vi "horn_coplanar.vi"(8 "Right points (world)":sgl[][](array[numeric]) format="%#.5f", 11 "Left points (lights)":sgl[][](array[numeric]) format="%#.5f") -> (2 "LR transform":T1)   [LabVIEW 2014]
uses:
  <vilib>/Analysis/Matrix/Datatypes/RealMatrix.ctl
  <vilib>/Analysis/baseanly.llb/Real Dot Product.vi
  <vilib>/Analysis/baseanly.llb/Real A x B.vi
  utilities/labview/norm_vec.vi
  <vilib>/Analysis/Matrix/Numeric/Conversions/Array To Matrix - RA.vi
  <vilib>/Analysis/NI_AALBase.lvlib
  <vilib>/Analysis/Matrix/NI_Matrix.lvlib
panel:
  # "Linear homogenous transform that maps the left points onto the right points."
  # "The input points, each row a point.   The points should be non-collinear and co-planar , which in practice only precisely applies when there are exactly three points.  This will give a reasonable result for > 3 points, but it will be not be a least-squares solution, being overly influenced by the first two points."
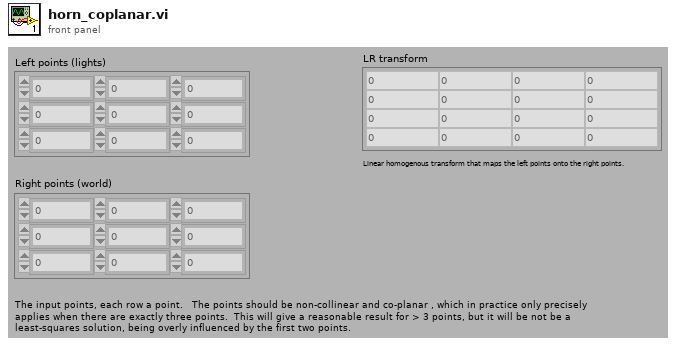
[diagram p1: front panel]
types:
  T1 = typedef "NI_Matrix.lvlib/RealMatrix.ctl" = dbl[][]
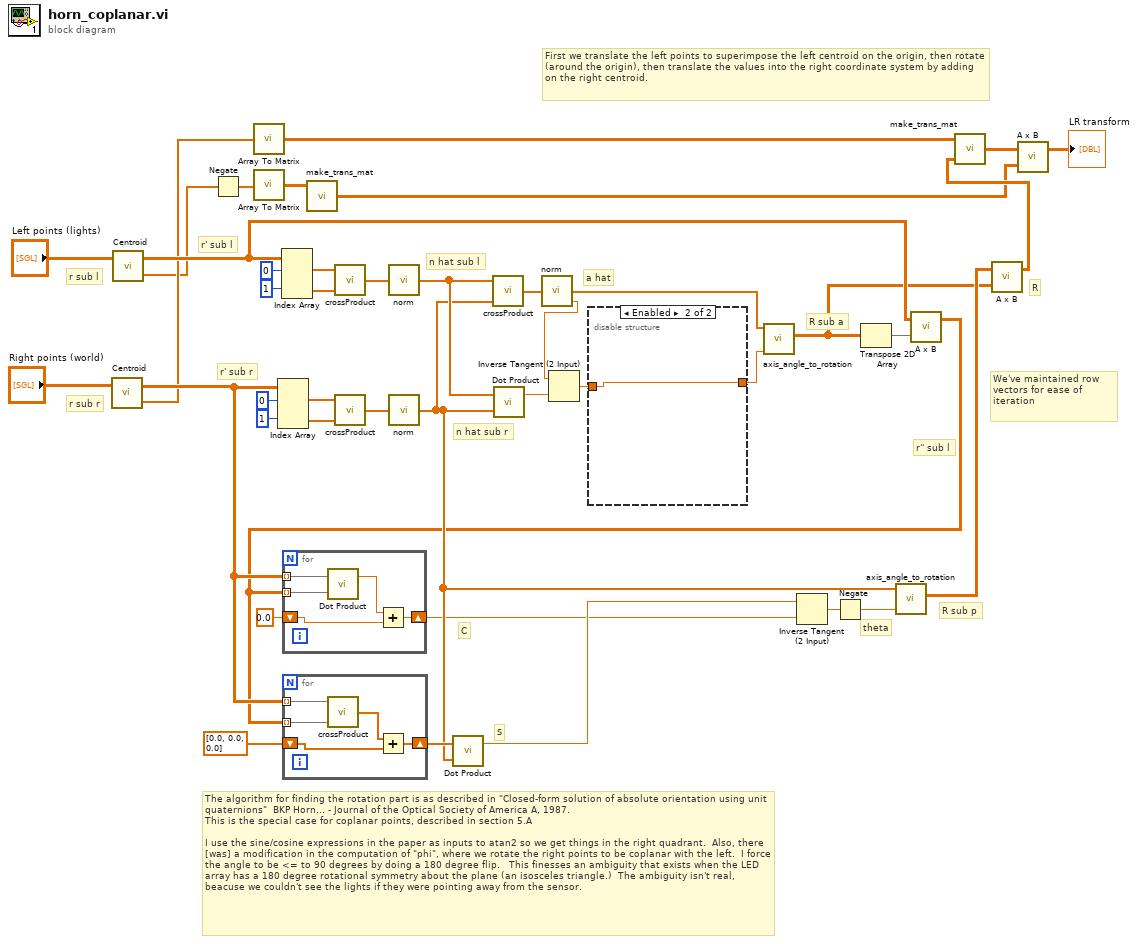
[diagram p0: block diagram]
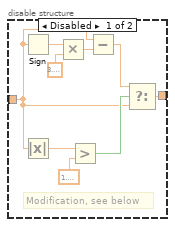
[diagram p2: hidden frame]
diagram:
  # "We've maintained row vectors for ease of iteration"
  # "First we translate the left points to superimpose the left centroid on the origin, then rotate (around the origin), then translate the values into the right coordinate system by adding on the right centroid."
  # "The algorithm for finding the rotation part is as described in \"Closed-form solution of absolute orientation using unit quaternions\"  BKP Horn… - Journal of the Optical Society of America A, 1987.\nThis is the special case for coplanar points, described in section 5.A\n\nI use the sine/cosine expressions in the paper as inputs to atan2 so we get things in the right quadrant.  Also, there [was] a modification in the computation of \"phi\", where we rotate the right points to be coplanar with the left.  I force the angle to be <= to 90 degrees by doing a 180 degree flip.   This finesses an ambiguity that exists when the LED array has a 180 degree rotational symmetry about the plane (an isosceles triangle.)  The ambiguity isn't real, beacuse we couldn't see the lights if they were pointing away from the sensor."
  # "R"
  # "R sub p"
  # "theta"
  # "S"
  # "C"
  # "r'' sub l"
  # "R sub a"
  # "r' sub r"
  # "r' sub l"
  # "r sub l"
  # "r sub r"
  # "a hat"
  # "n hat sub r"
  # "n hat sub l"
  n1 = call "Centroid.vi"("Points"="Right points (world)") -> ("Centroid"=w5:sgl[], "Offset vectors"=w24:sgl[][])  [unwired: 1 out]
  n2 = call "Centroid.vi"("Points"="Left points (lights)") -> ("Centroid"=w3:sgl[], "Offset vectors"=w26:sgl[][])  [unwired: 1 out]
  n3 = Negate(x=w3) -> (-x=w4:sgl[])
  n4 = call-poly <vilib>:"Array To Matrix.vi"("Real 1D Array"=w5) -> ("Real Matrix (Column Vector)"=w7:T1)
  n5 = call-poly <vilib>:"Array To Matrix.vi"("Real 1D Array"=w4) -> ("Real Matrix (Column Vector)"=w10:T1)
  n6 = Index Array(array=w24, index (row) #1=0 ("index"), index (row) #2=1 ("index")) -> (element #1=w32:sgl[], element #2=w31:sgl[])  [unwired: 2 in]
  n7 = Index Array(array=w26, index (row) #1=0 ("index"), index (row) #2=1 ("index")) -> (element #1=w38:sgl[], element #2=w37:sgl[])  [unwired: 2 in]
  n8 = call "make_trans_mat.vi"("Translation"=w10) -> ("Transform"=w8:T1)  [unwired: 1 in, 3 out]
  n9 = call "crossProduct.vi"("B"=w37, "A"=w38) -> ("A x B"=w36:dbl[])  [unwired: 3 out]
  n10 = call "crossProduct.vi"("B"=w31, "A"=w32) -> ("A x B"=w35:dbl[])  [unwired: 3 out]
  n11 = call-poly "norm.vi"("vector"=w36) -> ("normalized vector"=w29:dbl[])  [unwired: 4 out]
  n12 = call-poly "norm.vi"("vector"=w35) -> ("normalized vector"=w21:dbl[])  [unwired: 4 out]
  n13 = call "crossProduct.vi"("B"=w21, "A"=w29) -> ("A x B"=w30:dbl[])  [unwired: 3 out]
  n14 = call-poly <vilib>:"Dot Product.vi"("Y Vector"=w21, "X Vector"=w29) -> ("X * Y"=w12:dbl)  [unwired: 1 out]
  n15 = call-poly "norm.vi"("vector"=w30) -> ("magnitude"=w11:dbl, "normalized vector"=w28:dbl[])  [unwired: 3 out]
  n16 = Inverse Tangent (2 Input)(1:w12, 2:w11) -> (0:w1:dbl)
  n17 = disable-structure shown="Enabled" {
    disable-tunnel: [w49 w52] -> w2
    disable-tunnel: w1 -> [w47 w52]
    frame Disabled {
      # "Modification, see below"
      n18 = Sign(1:w47) -> (0:w48:dbl)
      n19 = Absolute Value(x=w47) -> (abs(x)=w51:dbl)
      n20 = Multiply(x=w48, y=3.141592653589793) -> (x*y=w46:dbl)
      n21 = Greater?(x=w51, y=1.5707963267948966) -> (0:w50:bool)
      n22 = Subtract(x=w47, y=w46) -> (x-y=w45:dbl)
      n23 = Select(t=w45, s=w50, f=w47) -> (s? t:f=w49:dbl)
    }
    frame Enabled {
    }
  }
  n24 = call "axis_angle_to_rotation.vi"("Angle"=w2, "Axis"=w28) -> ("Rotation"=w18:T1)  [unwired: 9 out]
  n25 = Transpose 2D Array(2D array=w18) -> (transposed array=w27:T1)
  n26 = call-poly <vilib>:"A x B.vi"("B"=w27, "A"=w26) -> ("A x B"=w20:T1)  [unwired: 1 out]
  n27 = for {
    tunnel: w20 -> [w56] mode=indexing
    tunnel: w24 -> [w57] mode=indexing
    shift-right: [w55] -> w13
    shift-left: 0.0 ("index") -> [w53]
    n28 = call-poly <vilib>:"Dot Product.vi"("Y Vector"=w56, "X Vector"=w57) -> ("X * Y"=w54:dbl)  [unwired: 1 out]
    n29 = Add(x=w54, y=w53) -> (x+y=w55:dbl)
  }
  n30 = for {
    tunnel: w20 -> [w59] mode=indexing
    tunnel: w24 -> [w60] mode=indexing
    shift-right: [w62] -> w22
    shift-left: dbl[] [0.0, 0.0, 0.0] ("x*y") -> [w61]
    n31 = call "crossProduct.vi"("B"=w59, "A"=w60) -> ("A x B"=w58:dbl[])  [unwired: 3 out]
    n32 = Add(x=w58, y=w61) -> (x+y=w62:dbl[])
  }
  n33 = call-poly <vilib>:"Dot Product.vi"("Y Vector"=w21, "X Vector"=w22) -> ("X * Y"=w16:dbl)  [unwired: 1 out]
  n34 = Inverse Tangent (2 Input)(1:w13, 2:w16) -> (0:w15:dbl)
  n35 = Negate(x=w15) -> (-x=w14:dbl)
  n36 = call "axis_angle_to_rotation.vi"("Angle"=w14, "Axis"=w21) -> ("Rotation"=w19:T1)  [unwired: 9 out]
  n37 = call-poly <vilib>:"A x B.vi"("B"=w18, "A"=w19) -> ("A x B"=w9:T1)  [unwired: 1 out]
  n38 = call "make_trans_mat.vi"("Rotation"=w9, "Translation"=w7) -> ("Transform"=w6:T1)  [unwired: 3 out]
  n39 = call-poly <vilib>:"A x B.vi"("B"=w8, "A"=w6) -> ("A x B"=→"LR transform":T1)  [unwired: 1 out]
